vi "Destroy Printf Event.vi"(8 "error in (no error)":errorcluster) -> (0 "error out":errorcluster)   [LabVIEW 2013, in "SET_Printf.lvlib" / "LV_Printf Core.lvclass"]
uses:
  LV_Printf Core.lvclass
  LV_Printf Core.lvclass/LV_Printf Core.ctl
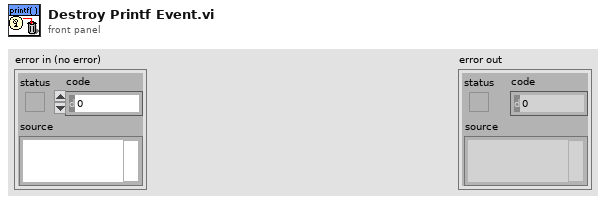
[diagram p1: front panel]
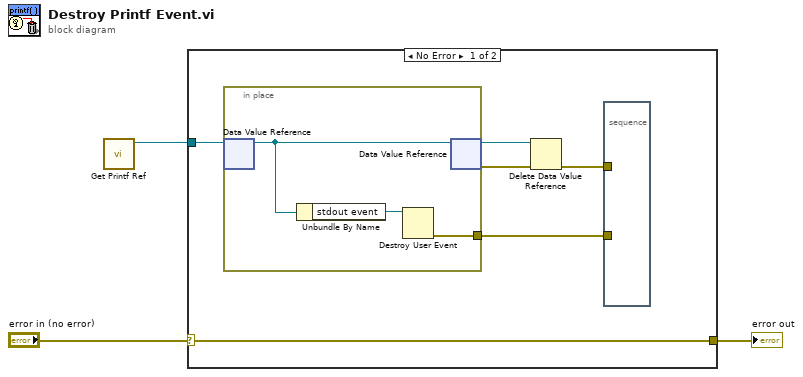
[diagram p0: block diagram]
diagram:
  n1 = call "Get Printf Ref.vi"() -> ("Printf DVR"=w1:refnum<data-value>)  [unwired: 11 in]
  n2 = case shown="No Error" "error in (no error)" {
    selector: "error in (no error)" -> [w7 w13]
    tunnel: [w7 w13] -> w2
    tunnel: w1 -> [w9 _]
    frame No Error {
      n3 = in-place {
        in-place-border: [w10] -> w5
        n4 = in-place-dvr #1(w9) -> (w12:refnum<class "LV_Printf Core.lvclass">)  [unwired: 1 out]
        n5 = Unbundle By Name(w12) -> ("stdout event"=w11:refnum<user-event>)
        n6 = Destroy User Event(user event=w11) -> (error out=w10:errorcluster)  [unwired: 1 in]
        n7 = in-place-dvr #1(w12) -> (w8:refnum<data-value>, w6:errorcluster)
      }
      n8 = Delete Data Value Reference(data value reference=w8, error in=w6) -> (error out=w4:errorcluster)  [unwired: 1 out]
      n9 = stacked-sequence {
        tunnel: w5 -> [_]
        tunnel: w4 -> [_]
        frame #0 {
        }
      }
    }
    frame Error {
    }
  }
  "error out" <- w2
